vi "WristToggle.vi"(1 "Step Control":bool, 2 "Vertical Control":bool, 3 "Horizontal Control":bool, 4 "Force State":i32) -> (0 "State":i32)   [LabVIEW 2014]
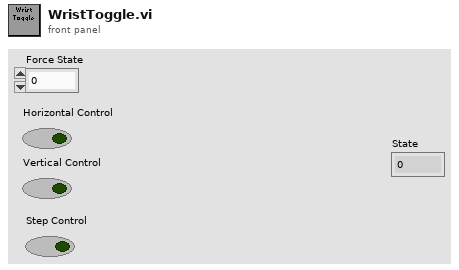
[diagram p1: front panel]
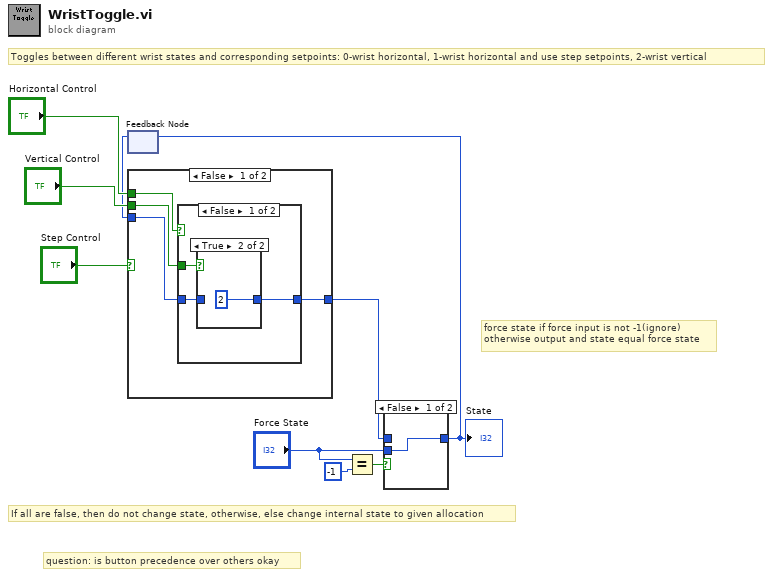
[diagram p0: block diagram]
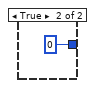
[diagram p4: hidden frame]
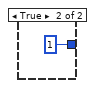
[diagram p5: hidden frame]
diagram:
  # "force state if force input is not -1(ignore)\notherwise output and state equal force state"
  # "question: is button precedence over others okay"
  # "If all are false, then do not change state, otherwise, else change internal state to given allocation"
  # "Toggles between different wrist states and corresponding setpoints: 0-wrist horizontal, 1-wrist horizontal and use step setpoints, 2-wrist vertical"
  n1 = feedback #1() -> (w6:i32)  [unwired: 1 in]
  n2 = case shown="False" "Step Control" {
    tunnel: "Horizontal Control" -> [w13 _]
    tunnel: "Vertical Control" -> [w12 _]
    tunnel: [w11 1] -> w5
    tunnel: w6 -> [w10 _]
    frame False {
      n3 = case shown="False" w13 {
        tunnel: w12 -> [w16 _]
        tunnel: [w15 0] -> w11
        tunnel: w10 -> [w14 _]
        frame False {
          n4 = case shown="True" w16 {
            tunnel: [w17 2] -> w15
            tunnel: w14 -> [w17 _]
            frame False {
            }
            frame True {
            }
          }
        }
        frame True {
        }
      }
    }
    frame True {
    }
  }
  n5 = Equal?(x="Force State", y=-1) -> (x = y?=w2:bool)
  n6 = case shown="False" w2 {
    tunnel: w5 -> [_ w22]
    tunnel: [w21 w22] -> w4
    tunnel: "Force State" -> [w21 _]
    frame False {
    }
    frame True {
    }
  }
  "State" <- w4
  n7 = feedback-in #1(w4) -> ()
